vi "logPublishPacket.vi"(9 "Timestamp (now)":timestamp, 10 "PUBLISH packet":refnum<class "PUBLISH.lvclass">) -> (2 "Publish Log":string)   [LabVIEW 2019]
uses:
  <vilib>/LabVIEW Open Source Project/MQTT Control Packets/Control Packets/PUBLISH/PUBLISH.lvclass
  <vilib>/LabVIEW Open Source Project/MQTT Control Packets/Control Packets/ControlPacket/ControlPacket.lvclass
  C:/Program Files (x86)/National Instruments/LabVIEW 2019/vi.lib/LabVIEW Open Source Project/MQTT Control Packets/Control Packets/ControlPacket/ControlPacket.lvclass
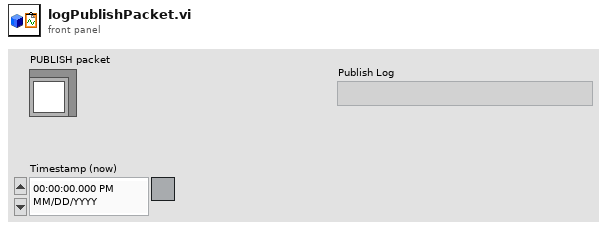
[diagram p1: front panel]
types:
  T1 = typedef "MQTT_Control_Packets.lvlib/ControlPacket.lvclass/QualityOfService -- enum.ctl" = enum16{"0 (At Most Once)", "1 (At Least Once)", "2 (Exactly Once)"}
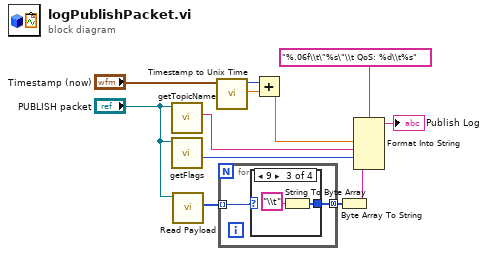
[diagram p0: block diagram]
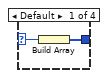
[diagram p2: hidden frame]
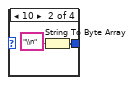
[diagram p3: hidden frame]
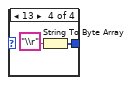
[diagram p4: hidden frame]
diagram:
  n1 = call <vilib>:"getTopicName.vi"("PUBLISH in"="PUBLISH packet") -> ("Topic"=w12:string)  [unwired: 8 in, 2 out]
  n2 = call-dynamic "getFlags.vi"("PUBLISH in"="PUBLISH packet") -> ("QoS"=w11:T1)  [unwired: 7 in, 3 out]
  n3 = call <vilib>:"Read Payload.vi"("ControlPacket in"="PUBLISH packet") -> ("Payload"=w6:u8[])  [unwired: 9 in, 1 out]
  n4 = call <vilib>:"Timestamp to Unix Time.vi"("Timestamp (now)"="Timestamp (now)") -> ("Fractional Second"=w8:dbl, "Unix Time (s)"=w9:i64)  [unwired: 9 in]
  n5 = for {
    tunnel: w6 -> [w14] mode=indexing
    tunnel: [w13] -> w5 mode=concatenating
    n6 = case shown="9" w14 {
      selector: w14 -> [w16 _ _ _]
      tunnel: [w15 w18 w20 w22] -> w13
      frame Default {
        n7 = Build Array(w16) -> (w15:u8[])
      }
      frame 10 {
        n8 = String To Byte Array(string="\\n") -> (unsigned byte array=w18:u8[])
      }
      frame 9 {
        n9 = String To Byte Array(string="\\t") -> (unsigned byte array=w20:u8[])
      }
      frame 13 {
        n10 = String To Byte Array(string="\\r") -> (unsigned byte array=w22:u8[])
      }
    }
  }
  n11 = Add(x=w9, y=w8) -> (x+y=w7:dbl)
  n12 = Byte Array To String(unsigned byte array=w5) -> (string=w10:string)
  n13 = Format Into String(format string="%.06f\\t\"%s\"\\t QoS: %d\\t%s", w7, w12, w11, w10) -> (resulting string=→"Publish Log":string)  [unwired: 2 in, 1 out]
